vi "HH_CheckErrorCode.vi"(0 "errcode":i32, 11 "error in (no error)":errorcluster) -> (4 "Is Error":bool, 15 "error out":errorcluster)   [LabVIEW 2013]
uses:
  Documents/Workspace/Labview_Workspace/CoreSetupNew/MT Scan/SubVIs/hhlib.dll
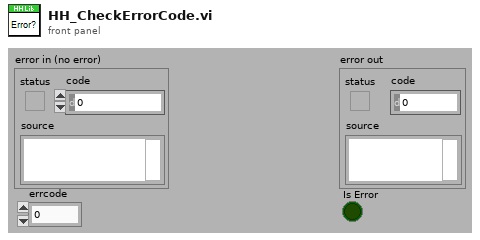
[diagram p1: front panel]
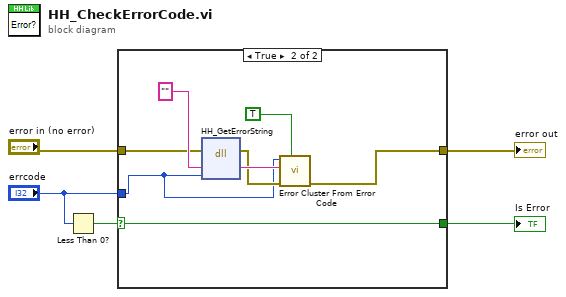
[diagram p0: block diagram]
diagram:
  n1 = Less Than 0?(x="errcode") -> (x < 0?=w3:bool)
  n2 = case shown="True" w3 {
    selector: w3 -> [w6 w9]
    tunnel: "error in (no error)" -> [w7 w12]
    tunnel: "errcode" -> [_ w11]
    tunnel: [w7 w10] -> w2
    tunnel: [w6 w9] -> w1
    frame False {
    }
    frame True {
      n3 = dll-call lib="C:/Users/dhaehnel/Documents/Workspace/Labview_Workspace/CoreSetupNew/MT Scan/SubVIs/hhlib.dll" fn="HH_GetErrorString"(error in=w12, "errstring"="", "errcode"=w11) -> (error out=w14:errorcluster, "errstring"=w15:string)  [unwired: 4 in, 1 out]
      n4 = call <vilib>:"Error Cluster From Error Code.vi"("show call chain? (False)"=TRUE, "error in (no error)"=w14, "error message (\"\")"=w15, "error code (0)"=w11) -> ("error out"=w10:errorcluster)  [unwired: 5 in]
    }
  }
  "error out" <- w2
  "Is Error" <- w1
